vi "Reset.vi"(8 "error in (no error)":errorcluster, 11 "NHRDCModel in":refnum<class "NHRDCPowerModel.lvclass">) -> (0 "error out":errorcluster, 3 "NHRDCModel out":refnum<class "NHRDCPowerModel.lvclass">)   [LabVIEW 2018, in "AcPwrPlugins.lvlib" / "NHRDCPowerModel.lvclass"]
doc: "This VI resets the instrument(s) into a know state."
uses:
  NHRDCPowerModel.lvclass
  AcPwrBaseClass/AcPwrBase.lvclass
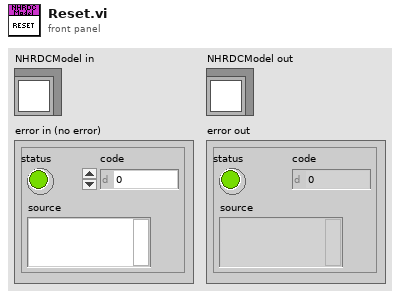
[diagram p1: front panel]
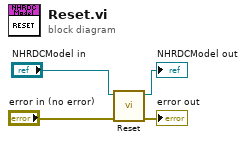
[diagram p0: block diagram]
diagram:
  n1 = call-parent "Reset.vi"("error in (no error)"="error in (no error)", "AcPwrBase in"="NHRDCModel in") -> ("error out"=→"error out":errorcluster, "AcPwrBase out"=→"NHRDCModel out":refnum<class "NHRDCPowerModel.lvclass">)  [unwired: 8 in]
